vi "Create Wrapper.vi"(9 "Alias":string, 10 "Actor":refnum<class "Actor.lvclass">) -> ()   [LabVIEW 2021, in "jettl.lvlib" / "jettl.lvclass"]
uses:
  jettl.lvclass
  Actor/Actor/Actor.lvclass
  C:/git/jettl/src/Actor/Actor/Actor.lvclass
  State/Destroy State/Destroy State.lvclass
  C:/git/jettl/src/jettl/State/State/State.lvclass
  jettl.lvclass/jettl.ctl
  jettl.lvlib
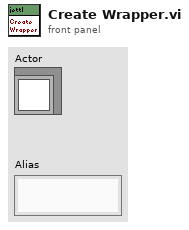
[diagram p1: front panel]
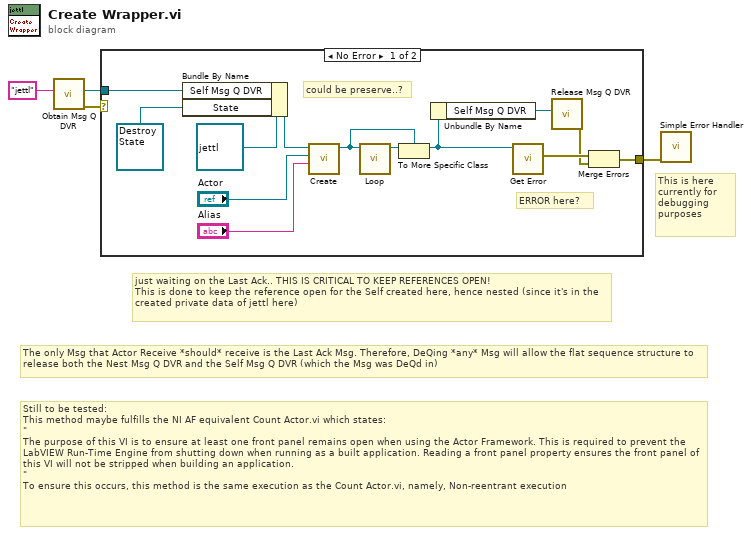
[diagram p0: block diagram]
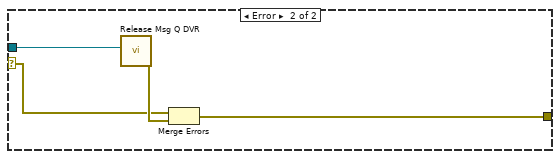
[diagram p2: hidden frame]
diagram:
  # "just waiting on the Last Ack.. THIS IS CRITICAL TO KEEP REFERENCES OPEN!\nThis is done to keep the reference open for the Self created here, hence nested (since it's in the created private data of jettl here)"
  # "Still to be tested:\nThis method maybe fulfills the NI AF equivalent Count Actor.vi which states:\n\"\nThe purpose of this VI is to ensure at least one front panel remains open when using the Actor Framework. This is required to prevent the LabVIEW Run-Time Engine from shutting down when running as a built application. Reading a front panel property ensures the front panel of this VI will not be stripped when building an application.\n\"\nTo ensure this occurs, this method is the same execution as the Count Actor.vi, namely, Non-reentrant execution"
  # "This is here currently for debugging purposes"
  # "The only Msg that Actor Receive *should* receive is the Last Ack Msg. Therefore, DeQing *any* Msg will allow the flat sequence structure to release both the Nest Msg Q DVR and the Self Msg Q DVR (which the Msg was DeQd in)"
  n1 = call "Obtain Msg Q DVR.vi"("Msg Q DVR Alias"="jettl") -> ("error out"=w2:errorcluster, "Msg Q DVR"=w4:refnum<data-value>)  [unwired: 9 in]
  n2 = case shown="No Error" w2 {
    selector: w2 -> [_ w18]
    tunnel: w4 -> [w16 w21]
    tunnel: [w15 w20] -> w3
    frame No Error {
      # "could be preserve..?"
      # "ERROR here?"
      n3 = Bundle By Name(cluster=refnum<class "jettl.lvclass"> refnum ("Self Actor in"), "Self Msg Q DVR"=w16, "State"=refnum<class "Destroy State.lvclass"> refnum ("jettl.lvlib:Destroy State.lvclass")) -> (w14:refnum<class "jettl.lvclass">)
      n4 = call-dynamic "Create.vi"("Alias"="Alias", "Actor"="Actor", "jettl in"=w14) -> ("jettl out"=w6:refnum<class "jettl.lvclass">)  [unwired: 8 in]
      n5 = call "Loop.vi"("Actor in"=w6) -> ("Actor out"=w7:refnum<class "Actor.lvclass">)  [unwired: 10 in]
      n6 = To More Specific Class(target class=w6, reference=w7) -> (specific class reference=w8:refnum<class "jettl.lvclass">)  [unwired: 1 in, 1 out]
      n7 = Unbundle By Name(w8) -> ("Self Msg Q DVR"=w17:refnum<data-value>)
      n8 = call-dynamic "Get Error.vi"("jettl in"=w8) -> ("Error"=w10:errorcluster)  [unwired: 10 in]
      n9 = call "Release Msg Q DVR.vi"("Msg Q DVR"=w17) -> ("error out"=w9:errorcluster)  [unwired: 10 in]
      n10 = Merge Errors(w10, w9) -> (w15:errorcluster)
    }
    frame Error {
      n11 = call "Release Msg Q DVR.vi"("Msg Q DVR"=w21) -> ("error out"=w19:errorcluster)  [unwired: 10 in]
      n12 = Merge Errors(w18, w19) -> (w20:errorcluster)
    }
  }
  n13 = call <vilib>:"Simple Error Handler.vi"("error in (no error)"=w3) -> ()  [unwired: 4 in, 5 out]
